vi "Get Database.vi"(8 "error in (no error)":errorcluster, 11 "Table Configuration Basic DB in":refnum<class "Table Configuration Basic DB.lvclass">) -> (0 "error out":errorcluster, 2 "Database":refnum<class "Database Interface.lvclass">, 3 "Table Configuration Basic DB out":refnum<class "Table Configuration Basic DB.lvclass">)   [LabVIEW 2020, in "Table.lvlib" / "Table Configuration Basic DB.lvclass"]
uses:
  Table Configuration Basic DB.lvclass
  Database Libraries/Database Interfaces/Database Interface Class/Database Interface.lvclass
  Table Configuration Basic DB.lvclass/Table Configuration Basic DB.ctl
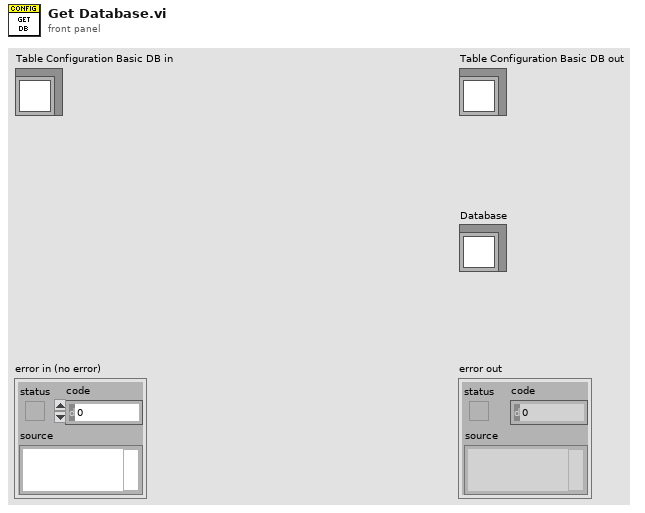
[diagram p1: front panel]
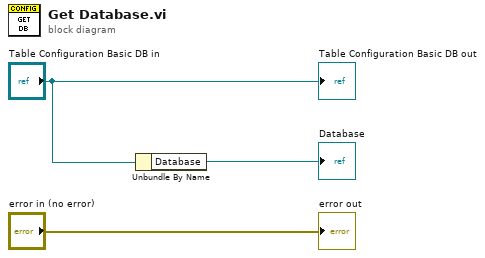
[diagram p0: block diagram]
diagram:
  n1 = Unbundle By Name("Table Configuration Basic DB in") -> ("Database"=→"Database":refnum<class "Database Interface.lvclass">)
  "error out" <- "error in (no error)"
  "Table Configuration Basic DB out" <- "Table Configuration Basic DB in"
